vi "Read Weighting (Population).vi"(8 "error in (no error)":errorcluster, 11 "Standard Averager in":refnum<class "Standard Averager.lvclass">) -> (0 "error out":errorcluster, 2 "Weighting (Population)":enum16{"Sample", "Population"}(ring)=enum."Population", 3 "Standard Averager out":refnum<class "Standard Averager.lvclass">)   [LabVIEW 2018, in "Standard Averager.lvclass"]
uses:
  Standard Averager.lvclass
  Standard Averager.lvclass/Standard Averager.ctl
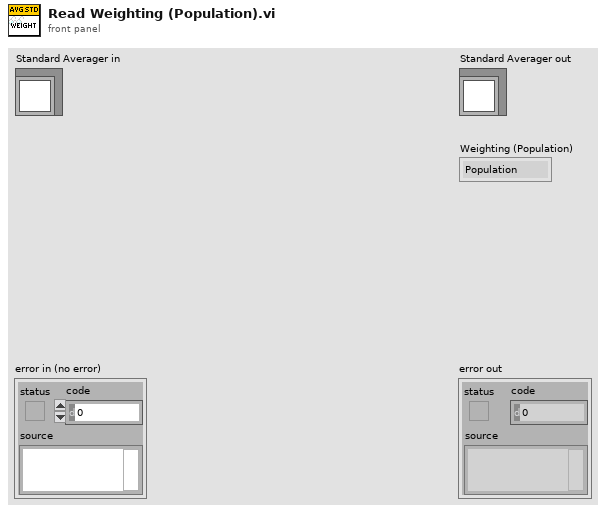
[diagram p1: front panel]
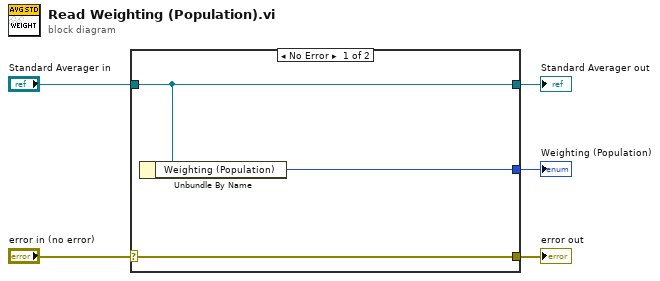
[diagram p0: block diagram]
diagram:
  n1 = case shown="No Error" "error in (no error)" {
    selector: "error in (no error)" -> [w8 w9]
    tunnel: [w8 w9] -> w4
    tunnel: [w7 w10] -> w2
    tunnel: "Standard Averager in" -> [w7 w10]
    tunnel: [w6 _] -> w1
    frame No Error {
      n2 = Unbundle By Name(w7) -> ("Weighting (Population)"=w6:enum16{"Sample", "Population"})
    }
    frame Error {
    }
  }
  "error out" <- w4
  "Standard Averager out" <- w2
  "Weighting (Population)" <- w1
